vi "Thorlabs-Clean pDataBuffer.vi"(1 "pDataBuffer in":u16[](array[numeric])) -> (0 "pDataBuffer out":u16[](array[numeric]))   [LabVIEW 2020]
uses:
  _Globals/Global Controls.vi
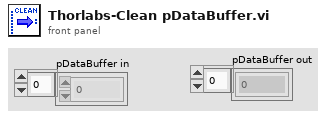
[diagram p1: front panel]
types:
  T1 = typedef "Confocal Controls.ctl" = cluster{"Channel Selection":enum32{"A", "B", "AB"}, "Pixel Count":cluster{"Pixels in X":u32, "Pixels in Y":u32}, "Field Size":dbl, "Frames":u8, "Averaging":bool, "Alignment":dbl, "Scan Mode":bool, "Gain":cluster{"Gain A":u8, "Gain B":u8}, "Enable PMTs":cluster{"A":bool, "B":bool}, "Voltage Range":cluster{"Range A":u16, "Range B":u16}, "Multi Frame Count":dbl, "Trigger Mode":dbl, "Real Time Averaging":bool, "PFOV":dbl, "MicronsPerPx":dbl}
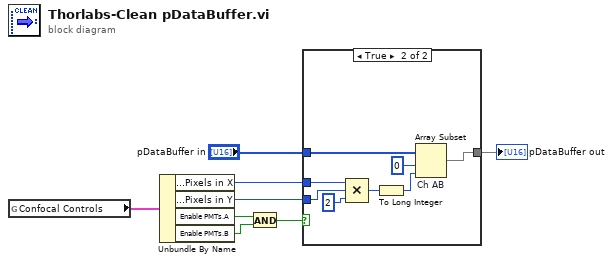
[diagram p0: block diagram]
diagram:
  n1 = global read "Global Controls.vi" "Confocal Controls"() -> (w6:T1)
  n2 = Unbundle By Name(w6) -> ("Pixel Count.Pixels in X"=w8:u32, "Pixel Count.Pixels in Y"=w7:u32, "Enable PMTs.A"=w5:bool, "Enable PMTs.B"=w4:bool)
  n3 = And(x=w5, y=w4) -> (x .and. y?=w3:bool)
  n4 = case shown="True" w3 {
    tunnel: w8 -> [_ w15]
    tunnel: w7 -> [_ w14]
    tunnel: "pDataBuffer in" -> [w9 w16]
    tunnel: [w9 w10] -> w1
    frame False {
    }
    frame True {
      n5 = Compound Arithmetic op=MULTIPLY(w15, w14, u32 2 ("value")) -> (w12:u32)
      n6 = To Long Integer(number=w12) -> (32bit integer=w11:i32)
      n7 = Array Subset "Ch AB"(array=w16, index=0, length=w11) -> (w10:u16[])
    }
  }
  "pDataBuffer out" <- w1
